vi "Compress String.vi"(8 "error in (no error)":errorcluster, 10 "String":string) -> (0 "error out":errorcluster, 2 "Compressed String":string)   [LabVIEW 2018, in "Kompress.lvlib"]
uses:
  Kompress.lvlib
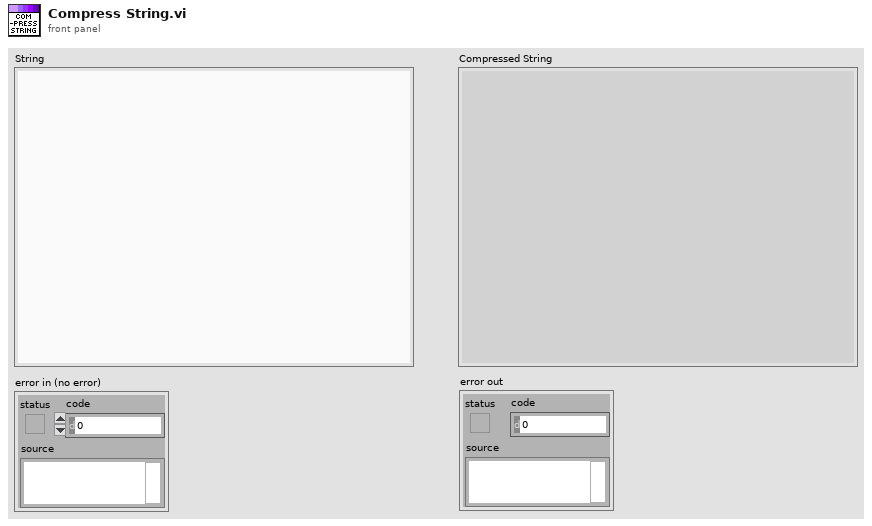
[diagram p1: front panel]
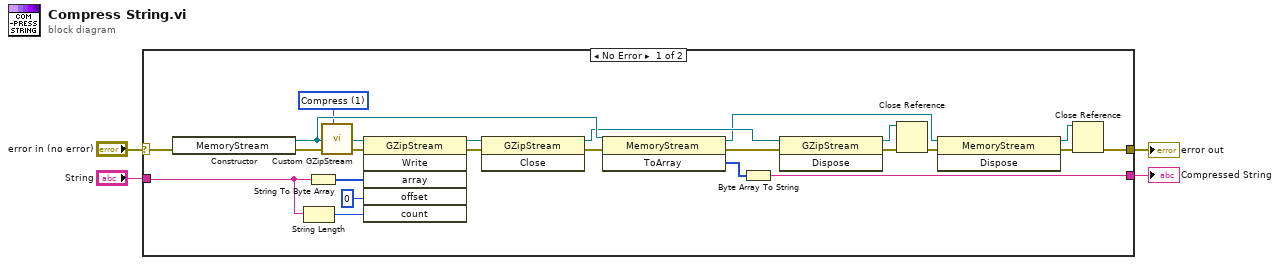
[diagram p0: block diagram]
diagram:
  n1 = case shown="No Error" "error in (no error)" {
    selector: "error in (no error)" -> [w6 w29]
    tunnel: "String" -> [w21 _]
    tunnel: [w16 _] -> w3
    tunnel: [w7 w29] -> w2
    frame No Error {
      w5 = 1 items=["Decompress", "Compress"] ("CompressionMode")
      n2 = constructor class="MemoryStream" ("mso")(error in=w6) -> (reference out=w22:refnum<k24>, error out=w25:errorcluster)  [unwired: 2 in, 1 out]
      n3 = String Length(string=w21) -> (length=w28:i32)
      n4 = String To Byte Array(string=w21) -> (unsigned byte array=w26:u8[])
      n5 = call "Custom GZipStream.vi"("Compression Mode"=w5, "System.IO.Stream"=w22, "error in (no error)"=w25) -> ("System.IO.Compression.GZipStream"=w23:refnum<k24>, "error out"=w24:errorcluster)  [unwired: 3 in]
      n6 = invoke class="GZipStream" method="Write"(reference=w23, error in=w24, "array"=w26, "offset"=0, "count"=w28) -> (reference out=w19:refnum<k24>, error out=w20:errorcluster)  [unwired: 1 in, 4 out]
      n7 = invoke class="GZipStream" method="Close"(reference=w19, error in=w20) -> (reference out=w9:refnum<k24>, error out=w18:errorcluster)  [unwired: 1 in, 1 out]
      n8 = invoke class="MemoryStream" method="ToArray"(reference=w22, error in=w18) -> (reference out=w8:refnum<k24>, error out=w15:errorcluster, "ToArray"=w17:u8[])  [unwired: 1 in]
      n9 = Byte Array To String(unsigned byte array=w17) -> (string=w16:string)
      n10 = invoke class="GZipStream" method="Dispose"(reference=w9, error in=w15) -> (reference out=w13:refnum<k24>, error out=w14:errorcluster)  [unwired: 1 in, 1 out]
      n11 = Close Reference(reference=w13, error in (no error)=w14) -> (error out=w12:errorcluster)
      n12 = invoke class="MemoryStream" method="Dispose"(reference=w8, error in=w12) -> (reference out=w10:refnum<k24>, error out=w11:errorcluster)  [unwired: 1 in, 1 out]
      n13 = Close Reference(reference=w10, error in (no error)=w11) -> (error out=w7:errorcluster)
    }
    frame Error {
    }
  }
  "error out" <- w2
  "Compressed String" <- w3
